vi "ex01_basics.vi"() -> ()   [LabVIEW 2019]
panel:
  out "Array 2":bool[](array[boolean])
  out "Array":i8[](array[knob]) scale=0.0..10.0
  out "Thermometer 5":i8(slide) scale=-100.0..80.0
  out "Thermometer 4":i32(slide) scale=-100.0..80.0
  out "Thermometer 3":u8(slide) scale=-100.0..80.0
  out "Thermometer 2":dbl(slide) scale=-100.0..80.0
  out "Thermometer":dbl(slide) scale=-100.0..80.0
  out "Tank":dbl(slide) scale=0.0..100.0
  in  "Knob":dbl(knob) scale=0.0..100.0
  in  "Button":bool
  in  "stop":bool
  out "LED":bool
  # "INC-KMUTT"
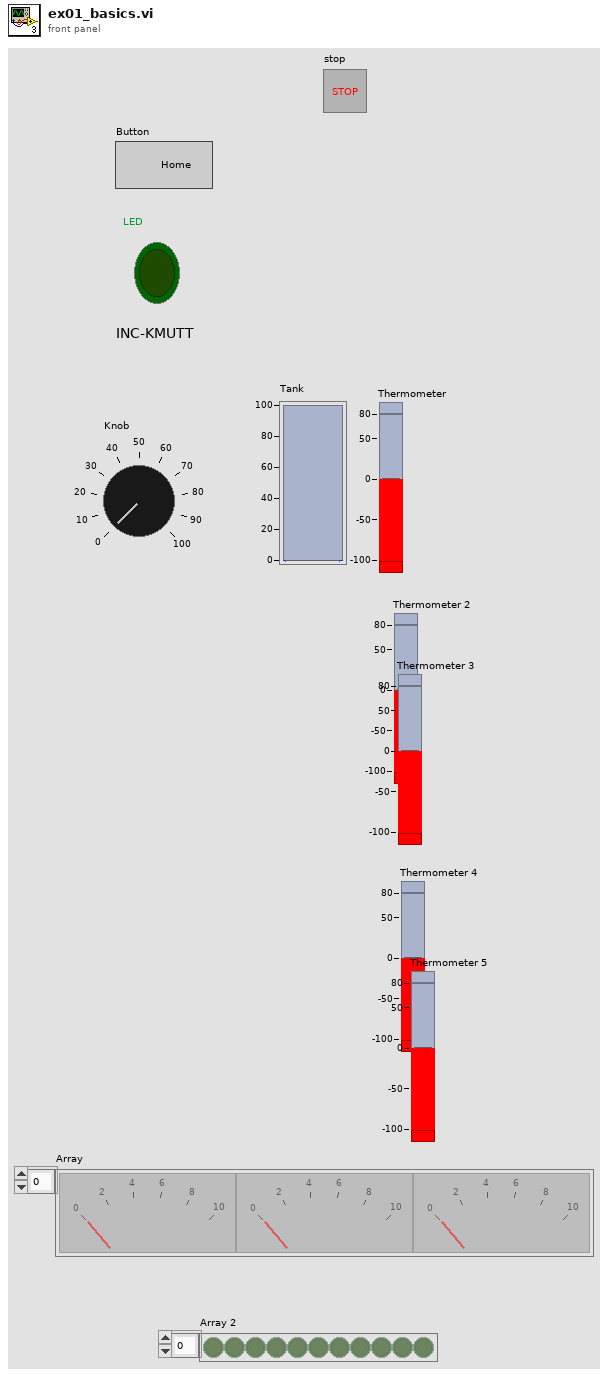
[diagram p1: front panel]
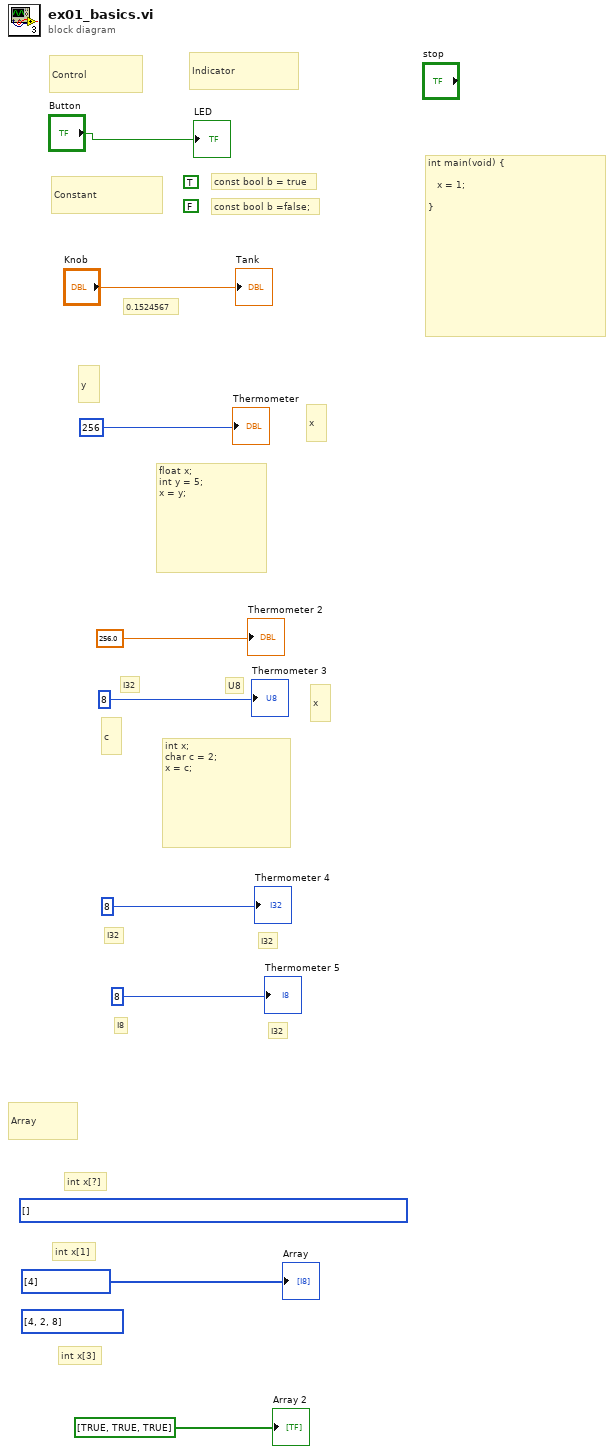
[diagram p0: block diagram]
diagram:
  (unwired) i8[] [4, 2, 8]
  (unwired) i8[] []
  (unwired) FALSE
  (unwired) TRUE
  # "int x[3]"
  # "int x[1]"
  # "int x[?]"
  # "Array"
  # "I32"
  # "I8"
  # "I32"
  # "I32"
  # "U8"
  # "I32"
  # "c"
  # "x"
  # "int x;\nchar c = 2;\nx = c;"
  # "x"
  # "y"
  # "float x;\nint y = 5;\nx = y;"
  # "0.1524567"
  # "int main(void) {\n\n   x = 1;\n\n}"
  # "const bool b =false;"
  # "const bool b = true"
  # "Constant"
  # "Indicator"
  # "Control"
  "LED" <- "Button"
  "Tank" <- "Knob"
  "Thermometer" <- 256
  "Thermometer 2" <- 256.0
  "Thermometer 3" <- 8
  "Thermometer 4" <- 8
  "Thermometer 5" <- i8 8
  "Array" <- i8[] [4]
  "Array 2" <- bool[] [TRUE, TRUE, TRUE]
